vi "UDP Named Service - Server.vi"() -> ()   [LabVIEW 2023]
doc: "Creates a named service and listens on the first available port. When a client connects to the service, it sends a response string to the client."
panel:
  in  "Message to Send":string="You are currently accessing UDP Named Service - Server.vi from client %s on port %d."
  in  "Stop":bool
  # "Overview: Demonstrates the use of the UDP functions to initialize a named UDP service that can send data to a client VI.\nInstructions:\n1. Run the VI.\n2. Open UDP Named Service - Client.vi and follow the instructions on its front panel.\n3. Click Stop to stop the VI."
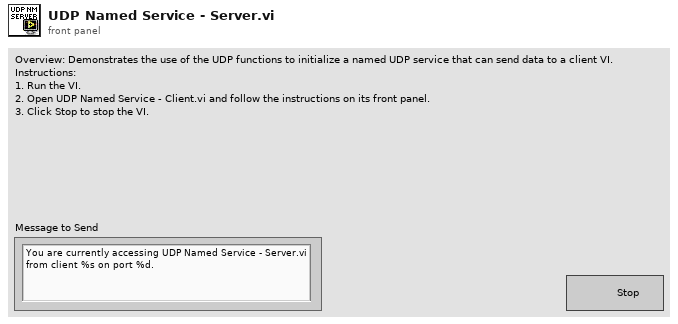
[diagram p1: front panel]
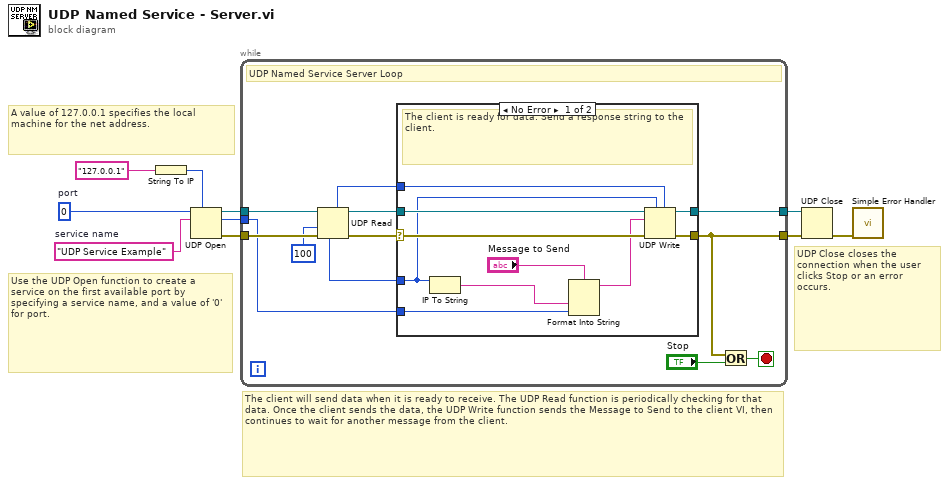
[diagram p0: block diagram]
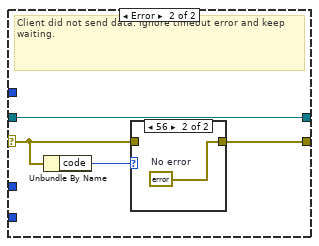
[diagram p2: hidden frame]
diagram:
  w1 = u16 0  # port
  w10 = "UDP Service Example"  # service name
  # "UDP Close closes the connection when the user clicks Stop or an error occurs."
  # "A value of 127.0.0.1 specifies the local machine for the net address."
  # "The client will send data when it is ready to receive. The UDP Read function is periodically checking for that data. Once the client sends the data, the UDP Write function sends the Message to Send to the client VI, then continues to wait for another message from the client."
  # "Use the UDP Open function to create a service on the first available port by specifying a service name, and a value of '0' for port."
  n1 = String To IP(1:"127.0.0.1") -> (0:w5:u32)
  n2 = UDP Open(7:w5, 10:w10, 11:w1) -> (port=w9:refnum<k16>, 0:w8:errorcluster, 2:w3:u16)  [unwired: 2 in]
  n3 = while {
    tunnel: [w13] -> w6
    tunnel: w9 -> [w22]
    tunnel: w8 -> [w18]
    tunnel: [w19] -> w7
    tunnel: w3 -> [w16]
    stop <- w15 stop-if-true
    # "UDP Named Service Server Loop"
    n4 = UDP Read(connection ID=w22, timeout ms (25000)=100, 8:w18) -> (error out=w21:errorcluster, 3:w20:refnum<k16>, 4:w17:u16, 6:w11:u32)  [unwired: 1 in, 1 out]
    n5 = case shown="No Error" w21 {
      selector: w21 -> [w32 w35]
      tunnel: w20 -> [w29 w36]
      tunnel: [w31 w33] -> w13
      tunnel: [w30 w36] -> w19
      tunnel: w11 -> [w27 _]
      tunnel: w17 -> [w28 _]
      tunnel: w16 -> [w25 _]
      frame No Error {
        # "The client is ready for data. Send a response string to the client."
        n6 = IP To String(2:w27) -> (0:w26:string)  [unwired: 1 in]
        n7 = Format Into String(format string="Message to Send", w26, w25) -> (resulting string=w23:string)  [unwired: 2 in, 1 out]
        n8 = UDP Write(address=w27, port or service name=w28, connection ID=w29, data in=w23, 8:w32) -> (error out=w31:errorcluster, 3:w30:refnum<k16>)  [unwired: 1 in]
      }
      frame Error {
        # "Client did not send data. Ignore timeout error and keep waiting."
        n9 = Unbundle By Name(w35) -> ("code"=w34:i32)
        n10 = case shown="56" w34 {
          tunnel: w35 -> [w37 _]
          tunnel: [w37 w38] -> w33
          frame Default {
          }
          frame 56 {
            w38 = errorcluster {"status"=FALSE, "code"=0, "source"=""}  # No error
          }
        }
      }
    }
    n11 = Or(x=w13, y="Stop") -> (x .or. y?=w15:bool)
  }
  n12 = UDP Close(connection ID=w7, 8:w6) -> (error out=w2:errorcluster)  [unwired: 1 out]
  n13 = call <vilib>:"Simple Error Handler.vi"("error in (no error)"=w2) -> ()  [unwired: 4 in, 5 out]
